vi "Garland_SB lambda demo.vi"() -> ()   [LabVIEW 2013]
panel:
  out "Tug Nav Data":cluster{"y":i32, "y":i32}
  out "Valid ?":bool
  out "error out":errorcluster
  out "UDP Time Out?":bool
  out "data rec'd":string="$,G,43,13,230,P,10,20,120,T,10,10,330,L,14,36,110,A,3,5,B,7,8,C,16,20,D,-1,-1,S,08,12,234\r"
  in  "stop":bool
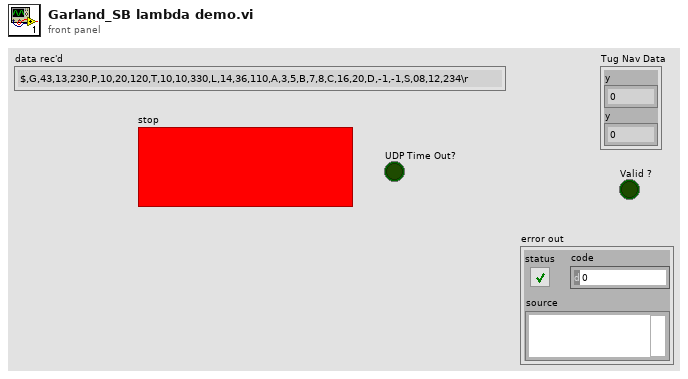
[diagram p1: front panel]
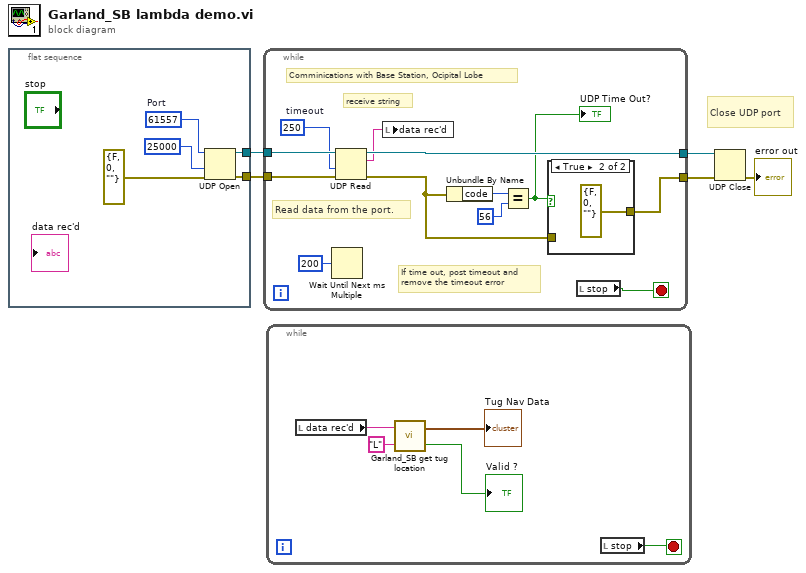
[diagram p0: block diagram]
diagram:
  # "Close UDP port"
  n1 = flat-sequence {
    tunnel: [w8] -> w3
    tunnel: [w7] -> w2
    frame #0 {
      w10 = u16 61557  # Port
      n2 = UDP Open(8:errorcluster {"status"=FALSE, "code"=0, "source"=""} ("error in (no error)"), 9:25000 ("timeout ms (25000)"), 11:w10) -> (port=w8:refnum<k16>, 0:w7:errorcluster)  [unwired: 2 in, 1 out]
    }
  }
  n3 = while {
    tunnel: w2 -> [w22]
    tunnel: w3 -> [w21]
    tunnel: [w20] -> w5
    tunnel: [w15] -> w4
    stop <- w11 stop-if-true
    w14 = 250  # timeout
    # "Comminications with Base Station, Ocipital Lobe"
    # "receive string"
    # "If time out, post timeout and\nremove the timeout error"
    # "Read data from the port."
    n4 = Wait Until Next ms Multiple(millisecond multiple=u32 200) -> ()  [unwired: 1 out]
    n5 = UDP Read(connection ID=w21, timeout ms (25000)=w14, 8:w22) -> (data out=w13:string, error out=w16:errorcluster, 3:w20:refnum<k16>)  [unwired: 1 in, 2 out]
    n6 = local write "data rec'd"(w13) -> ()
    n7 = Unbundle By Name(w16) -> ("code"=w19:i32)
    n8 = Equal?(x=w19, y=56) -> (x = y?=w17:bool)
    "UDP Time Out?" <- w17
    n9 = case shown="True" w17 {
      tunnel: [w23 errorcluster {"status"=FALSE, "code"=0, "source"=""} ("error out")] -> w15
      tunnel: w16 -> [w23 _]
      frame False {
      }
      frame True {
      }
    }
    n10 = local read "stop"() -> (w11:bool)
  }
  n11 = while {
    stop <- w29 stop-if-true
    n12 = local read "data rec'd"() -> (w28:string)
    n13 = call "Garland_SB get tug location.vi"("Tug"="L", "Nav String"=w28) -> ("Valid ?"=→"Valid ?":bool, "Tug Nav Data"=→"Tug Nav Data":cluster{"y":i32, "y":i32})
    n14 = local read "stop"() -> (w29:bool)
  }
  n15 = UDP Close(connection ID=w5, 8:w4) -> (error out=→"error out":errorcluster)  [unwired: 1 out]
